vi "NHRdischargechargetest.vi"() -> ()   [LabVIEW 2020]
uses:
  <instrlib>/NH Research Regenerative Test Series/Public/Configure/Output Safety.ctl
  <instrlib>/NH Research Regenerative Test Series/Public/Data/Read (Ave Current).vi
  <instrlib>/NH Research Regenerative Test Series/Public/Data/Low Level/Fetch (Ave Voltage).vi
  <instrlib>/NH Research Regenerative Test Series/Public/Data/Low Level/Fetch (Ave True Power).vi
  <instrlib>/NH Research Regenerative Test Series/NH Research Regenerative Test Series.lvlib
panel:
  out "String":string
  out "Status Byte Register":T1
  out "Ave True Power (W)":dbl
  out "Ave Voltage (V)":dbl
  out "Ave Current (A)":dbl
  in  "Logical Instrument Number":u32=1
  in  "stop":bool
  in  "Enable":T2
  in  "Resistance Setpoint (0 Ohms)":dbl format="%#.6g"
  in  "Power Setpoint (0 W)":dbl format="%#.6g"
  in  "Current Setpoint (0 A)":dbl format="%#.6g"
  in  "Voltage Setpoint (0 V)":dbl format="%#.6g"
  in  "Mode (0: Off)":i32(ring) items=["Off", "Standby", "Charge", "Discharge", "Battery"]
  in  "Battery Detect Voltage (0V)":dbl format="%#.6g"
  in  "Output Safety":T3
  in  "VISA resource name":refnum<visa-resource-name>
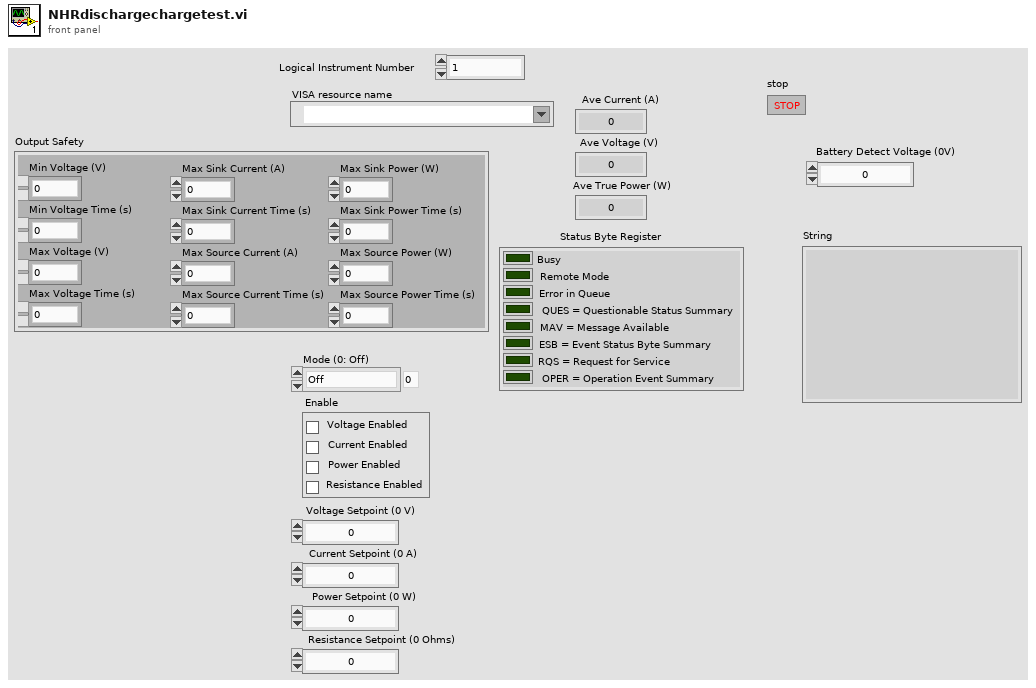
[diagram p1: front panel]
types:
  T1 = cluster{"Busy":bool, "Remote Mode":bool, "Error in Queue":bool, "QUES = Questionable Status Summary":bool, "MAV = Message Available":bool, "ESB = Event Status Byte Summary":bool, "RQS = Request for Service":bool, "OPER = Operation Event Summary":bool}
  T2 = cluster{"Voltage Enabled":bool, "Current Enabled":bool, "Power Enabled":bool, "Resistance Enabled":bool}
  T3 = typedef "NH Research Regenerative Test Series.lvlib/Output Safety.ctl" = cluster{"Min Voltage (V)":dbl, "Min Voltage Time (s)":dbl, "Max Voltage (V)":dbl, "Max Voltage Time (s)":dbl, "Max Sink Current (A)":dbl, "Max Sink Current Time (s)":dbl, "Max Source Current (A)":dbl, "Max Source Current Time (s)":dbl, "Max Sink Power (W)":dbl, "Max Sink Power Time (s)":dbl, "Max Source Power (W)":dbl, "Max Source Power Time (s)":dbl}
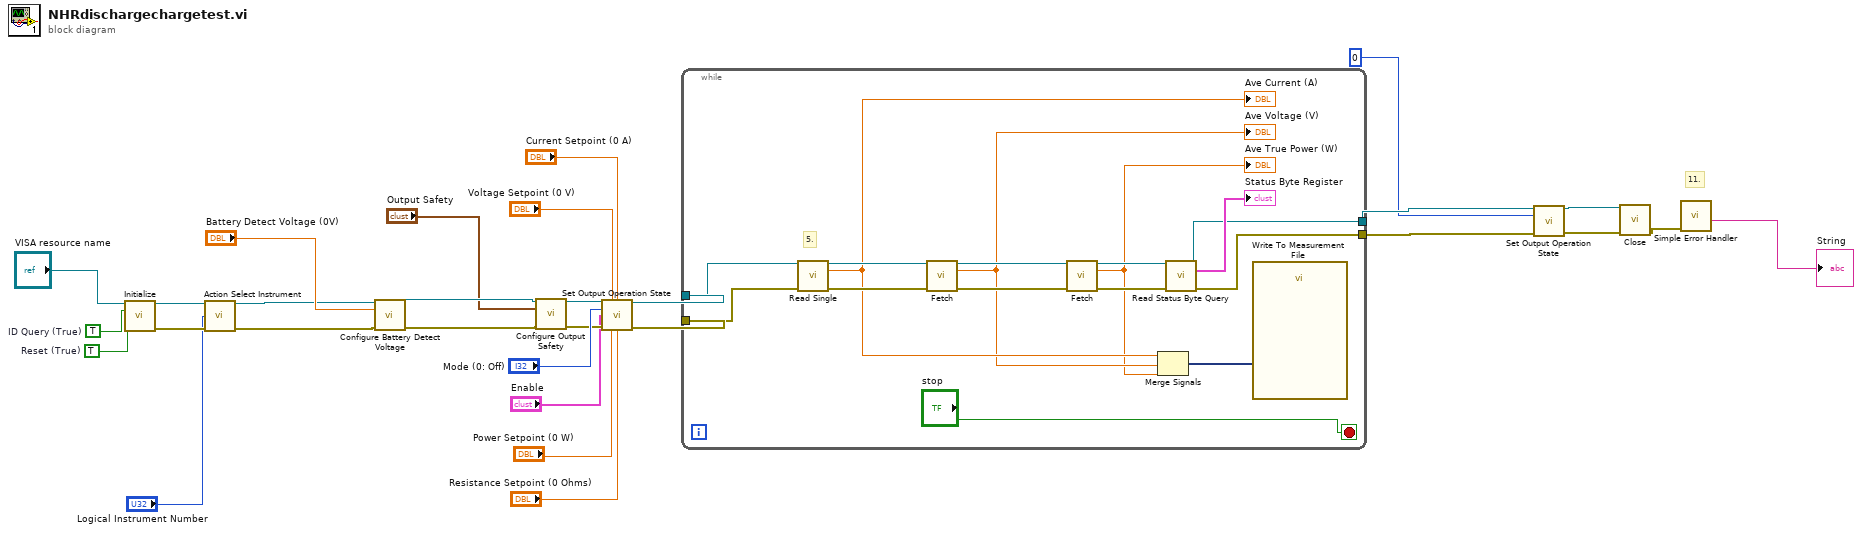
[diagram p0: block diagram]
diagram:
  w3 = TRUE  # ID Query (True)
  w2 = TRUE  # Reset (True)
  # "11."
  n1 = call <vilib>:"Initialize.vi"("VISA resource name"="VISA resource name", "ID Query (True)"=w3, "Reset (True)"=w2) -> ("VISA resource name out"=w7:refnum<visa-resource-name>, "error out"=w6:errorcluster)  [unwired: 11 in]
  n2 = call <instrlib>:"Action Select Instrument.vi"("VISA resource name"=w7, "Logical Instrument Number"="Logical Instrument Number", "error in (no error)"=w6) -> ("VISA resource name out"=w9:refnum<visa-resource-name>, "error out"=w8:errorcluster)  [unwired: 11 in]
  n3 = call <vilib>:"Configure Battery Detect Voltage.vi"("VISA resource name"=w9, "Battery Detect Voltage (0V)"="Battery Detect Voltage (0V)", "error in (no error)"=w8) -> ("VISA resource name out"=w28:refnum<visa-resource-name>, "error out"=w27:errorcluster)  [unwired: 11 in]
  n4 = call <vilib>:"Configure Output Safety.vi"("VISA resource name"=w28, "Output Safety"="Output Safety", "error in (no error)"=w27) -> ("VISA resource name out"=w23:refnum<visa-resource-name>, "error out"=w22:errorcluster)  [unwired: 11 in]
  n5 = call <vilib>:"Set Output Operation State.vi"("VISA resource name"=w23, "Voltage Setpoint (0 V)"="Voltage Setpoint (0 V)", "Current Setpoint (0 A)"="Current Setpoint (0 A)", "Mode (0: Off)"="Mode (0: Off)", "Enable"="Enable", "error in (no error)"=w22, "Power Setpoint (0 W)"="Power Setpoint (0 W)", "Resistance Setpoint (0 Ohms)"="Resistance Setpoint (0 Ohms)") -> ("VISA resource name out"=w21:refnum<visa-resource-name>, "error out"=w20:errorcluster)  [unwired: 6 in]
  n6 = while {
    tunnel: w21 -> [w37]
    tunnel: w20 -> [w36]
    tunnel: [w34] -> w14
    tunnel: [w33] -> w13
    stop <- "stop" stop-if-true
    # "5."
    n7 = call-poly <instrlib>:"Read Single.vi"("VISA resource name"=w37, "error in (no error)"=w36) -> ("VISA resource name out"=w42:refnum<visa-resource-name>, "Ave Current (A)"=w32:dbl, "error out"=w43:errorcluster)  [unwired: 11 in]
    "Ave Current (A)" <- w32
    n8 = call-poly <instrlib>:"Fetch.vi"("VISA resource name"=w42, "error in (no error)"=w43) -> ("VISA resource name out"=w41:refnum<visa-resource-name>, "Ave Voltage (V)"=w31:dbl, "error out"=w40:errorcluster)  [unwired: 11 in]
    "Ave Voltage (V)" <- w31
    n9 = call-poly <instrlib>:"Fetch.vi"("VISA resource name"=w41, "error in (no error)"=w40) -> ("VISA resource name out"=w39:refnum<visa-resource-name>, "Ave True Power (W)"=w30:dbl, "error out"=w38:errorcluster)  [unwired: 11 in]
    "Ave True Power (W)" <- w30
    n10 = Merge Signals "Merge Signals"(w32, w31, w30) -> (w45:dynamicdata)
    n11 = call <instrlib>:"Read Status Byte Query.vi"("VISA resource name"=w39, "error in (no error)"=w38) -> ("VISA resource name out"=w34:refnum<visa-resource-name>, "Status Byte Register"=→"Status Byte Register":T1, "error out"=w33:errorcluster)  [unwired: 11 in]
    n12 = call "Write To Measurement File"("Signals"=w45) -> ()  [unwired: 16 in, 3 out]
  }
  n13 = call <vilib>:"Set Output Operation State.vi"("VISA resource name"=w14, "Mode (0: Off)"=0, "error in (no error)"=w13) -> ("VISA resource name out"=w11:refnum<visa-resource-name>, "error out"=w10:errorcluster)  [unwired: 11 in]
  n14 = call <instrlib>:"Close.vi"("VISA resource name"=w11, "error in (no error)"=w10) -> ("error out"=w4:errorcluster)  [unwired: 13 in]
  n15 = call <vilib>:"Simple Error Handler.vi"("error in (no error)"=w4) -> ("source out"=→"String":string)  [unwired: 4 in, 4 out]
